vi "PXDAC4800_DisconnectToDeviceXD48.vi"(1 "Handle":i32) -> (0 "Status":i32)   [LabVIEW 2016]
uses:
  PXDAC4800.dll
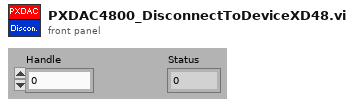
[diagram p1: front panel]
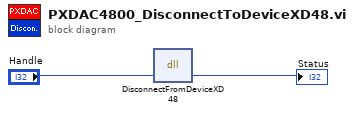
[diagram p0: block diagram]
diagram:
  n1 = dll-call lib="PXDAC4800.dll" fn="DisconnectFromDeviceXD48"("Handle"="Handle") -> (→"Status":i32)  [unwired: 4 in, 2 out]
